vi "FPGA Global Variables.vi"() -> ()   [LabVIEW 2016]
panel:
  out "FPGA Refnum":refnum<k20>
  out "FPGA VI Reference Out":refnum<k20>
  in  "Number Of Averages":u32=16
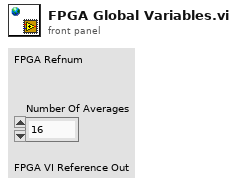
[diagram p1: front panel]
diagram:
